vi "Write Adapt To Source.vi"(8 "error in (no error)":errorcluster, 10 "AdaptToSource":bool, 11 "Numeric.lvclass in":refnum<class "Numeric.lvclass">) -> (0 "error out":errorcluster, 3 "Numeric.lvclass out":refnum<class "Numeric.lvclass">)   [LabVIEW 2015, in "Numeric.lvclass"]
uses:
  Numeric.lvclass
  Numeric.lvclass/Numeric.ctl
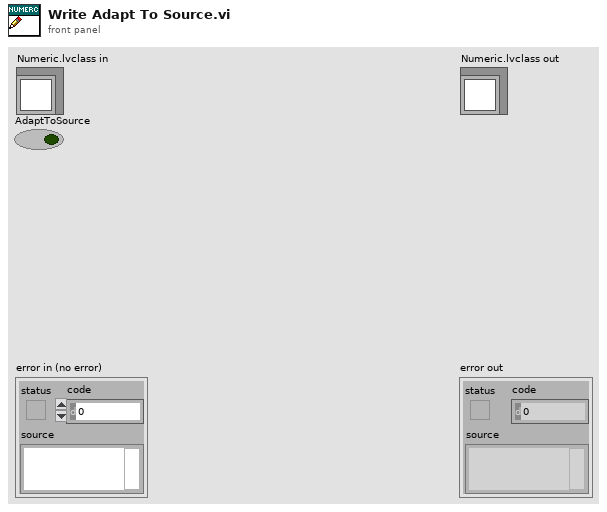
[diagram p1: front panel]
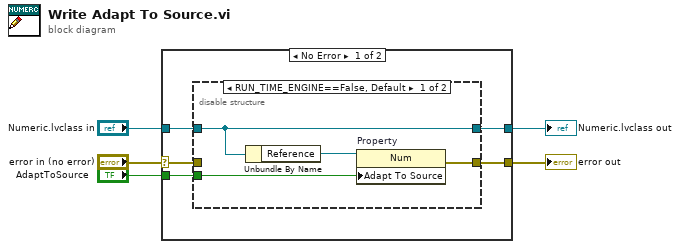
[diagram p0: block diagram]
diagram:
  n1 = case shown="No Error" "error in (no error)" {
    selector: "error in (no error)" -> [w6 w18]
    tunnel: [w10 w18] -> w4
    tunnel: [w7 w17] -> w2
    tunnel: "Numeric.lvclass in" -> [w8 w17]
    tunnel: "AdaptToSource" -> [w9 _]
    frame No Error {
      n2 = disable-structure shown="RUN_TIME_ENGINE==False, Default" {
        disable-tunnel: [w14 w15] -> w10
        disable-tunnel: w9 -> [w13 _]
        disable-tunnel: w8 -> [w11 w16]
        disable-tunnel: [w11 w16] -> w7
        disable-tunnel: w6 -> [_ w15]
        frame condition #0 (active) {
          n3 = Unbundle By Name(w11) -> ("Reference"=w12:refnum<vi>)
          n4 = property on="Property" class="Num"(reference=w12, "Adapt To Source"=w13) -> (error out=w14:errorcluster)  [unwired: 1 in, 1 out]
        }
        frame condition #1 {
        }
      }
    }
    frame Error {
    }
  }
  "error out" <- w4
  "Numeric.lvclass out" <- w2
